vi "GetParam.vi"(8 "error in (no error)":errorcluster caption="entrée d'erreur (pas d'erreur)", 11 "Label_Ranking_Loss.lvclass":refnum<class "Label_Ranking_Loss.lvclass">) -> (0 "error out":errorcluster caption="sortie d'erreur", 2 "label_ranking_loss":cluster{"sample_weight":dbl[]}, 3 "Label_Ranking_Loss.lvclass":refnum<class "Label_Ranking_Loss.lvclass">)   [LabVIEW 2020, in "Label_Ranking_Loss.lvclass"]
doc: "Get Parameters"
uses:
  Label_Ranking_Loss.lvclass
  Label_Ranking_Loss.lvclass/Label_Ranking_Loss.ctl
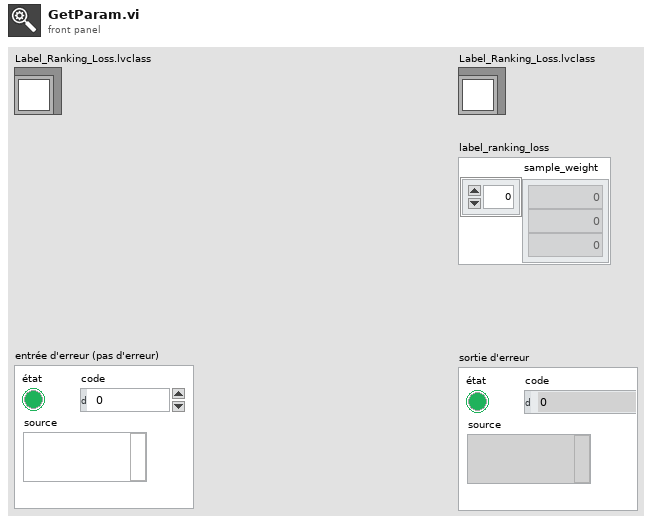
[diagram p1: front panel]
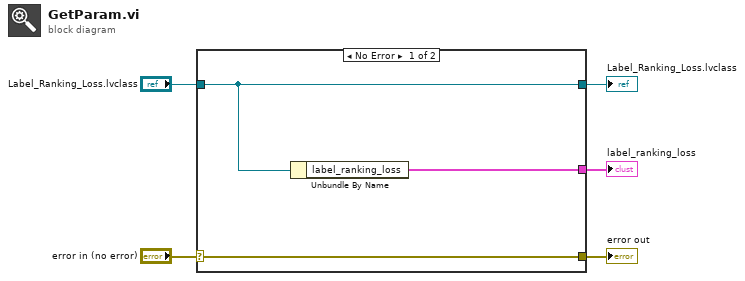
[diagram p0: block diagram]
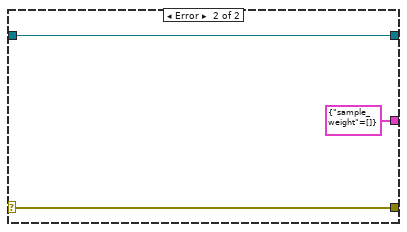
[diagram p2: hidden frame]
diagram:
  n1 = case shown="No Error" "error in (no error)" {
    selector: "error in (no error)" -> [w8 w10]
    tunnel: [w8 w10] -> w4
    tunnel: [w7 w11] -> w2
    tunnel: "Label_Ranking_Loss.lvclass" -> [w7 w11]
    tunnel: [w6 cluster{"sample_weight":dbl[]} {"sample_weight"=[]} ("label_ranking_loss")] -> w1
    frame No Error {
      n2 = Unbundle By Name(w7) -> ("label_ranking_loss"=w6:cluster{"sample_weight":dbl[]})
    }
    frame Error {
    }
  }
  "error out" <- w4
  "Label_Ranking_Loss.lvclass" <- w2
  "label_ranking_loss" <- w1
